vi "VI_X.vi"() -> ()   [LabVIEW 2015]
uses:
  <vilib>/vision/Vision Builder AI/API.llb/IVB Interface - VBAI Version.ctl
panel:
  out "COMMENTS":string
  in  "TOTAL NUMBER OF BRANCHS":i16=16
  out "INSPECTED IMAGE":T1(plugin-control)
  out "STATE TEST":bool
  out "INSPECTION NAME":string
  in  "error in 2":errorcluster
  out "error out 2":errorcluster
  out "INSPECTION PATH":path
  in  "ACTION":T2(ring)
  out "SESSION NAME":string
  in  "Number of Branch X":i16 caption="NUMBER OF BRANCH X" min=0
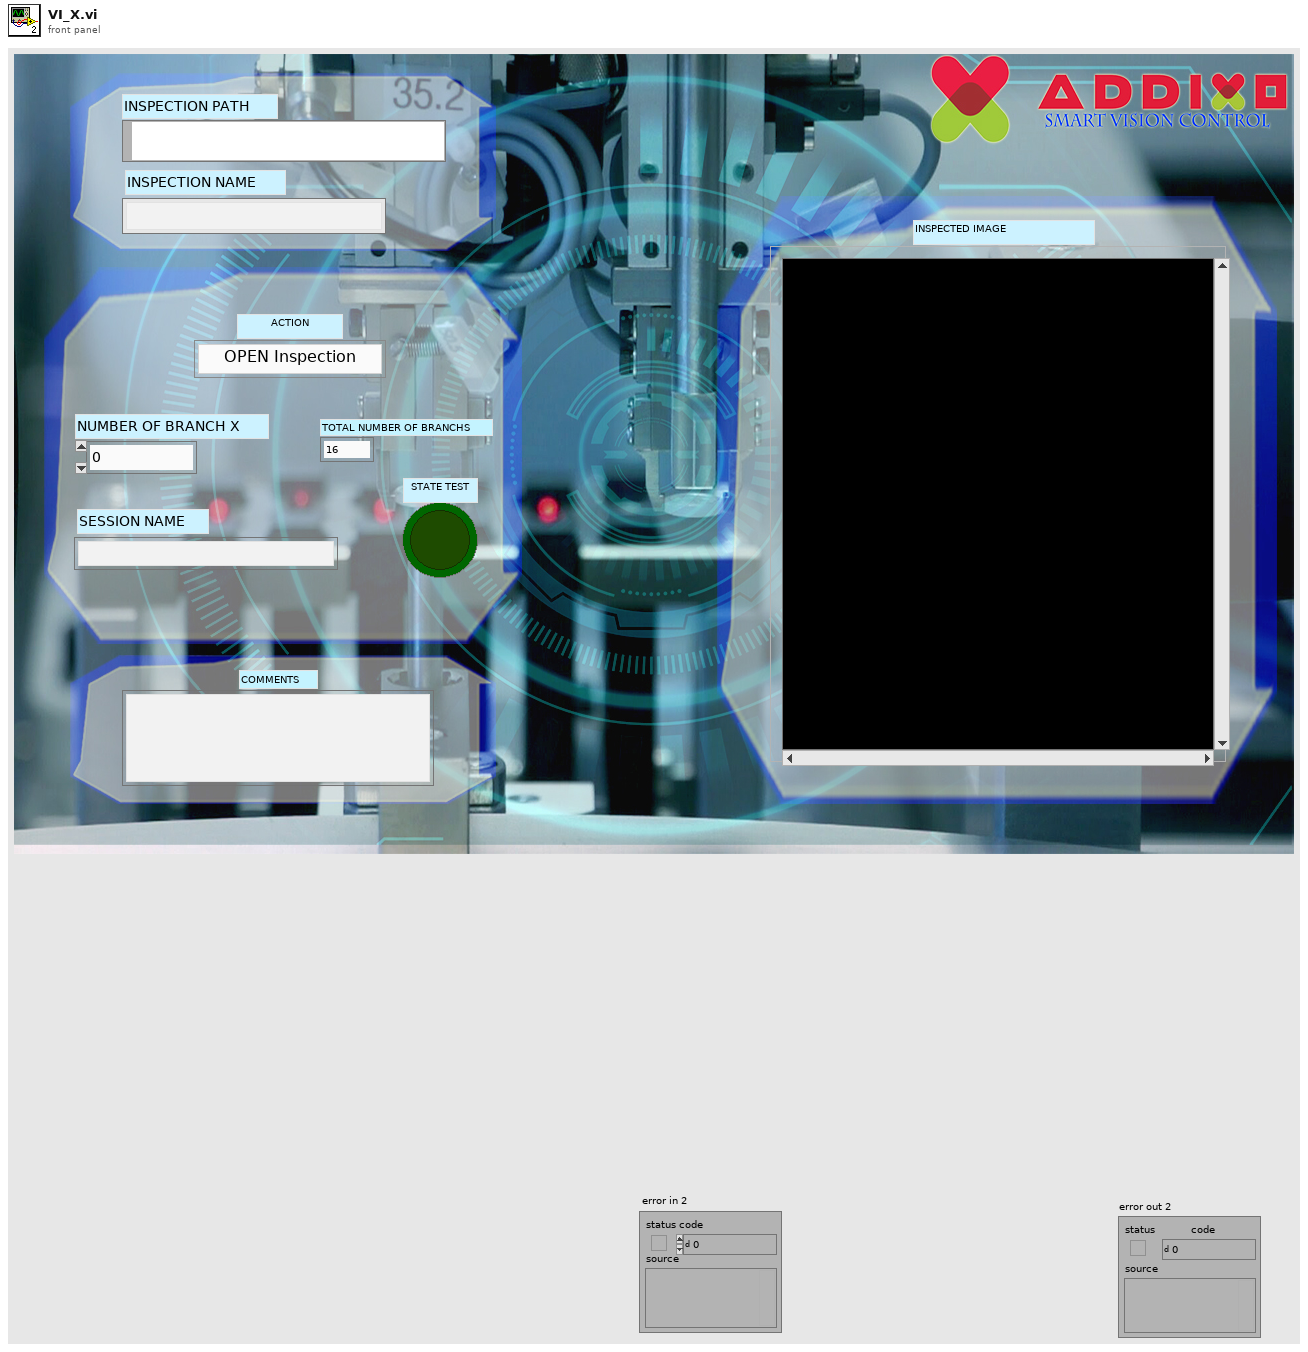
[diagram p1: front panel]
types:
  T1 = typedef "IMAQ Image.ctl" = refnum<image>
  T2 = enum16{"OPEN Inspection", "START Inspection", "Inspect", "CLOSE Inspection"}
  T3 = cluster{"PASS/FAIL Flag":bool, "Numeric Measurement":dbl, "String Measurement":string, "Report Text":string}
  T4 = typedef "IVB Interface - VBAI Version.ctl" = u16
  T5 = typedef "VBAIInterface.ctl" = refnum<k21>
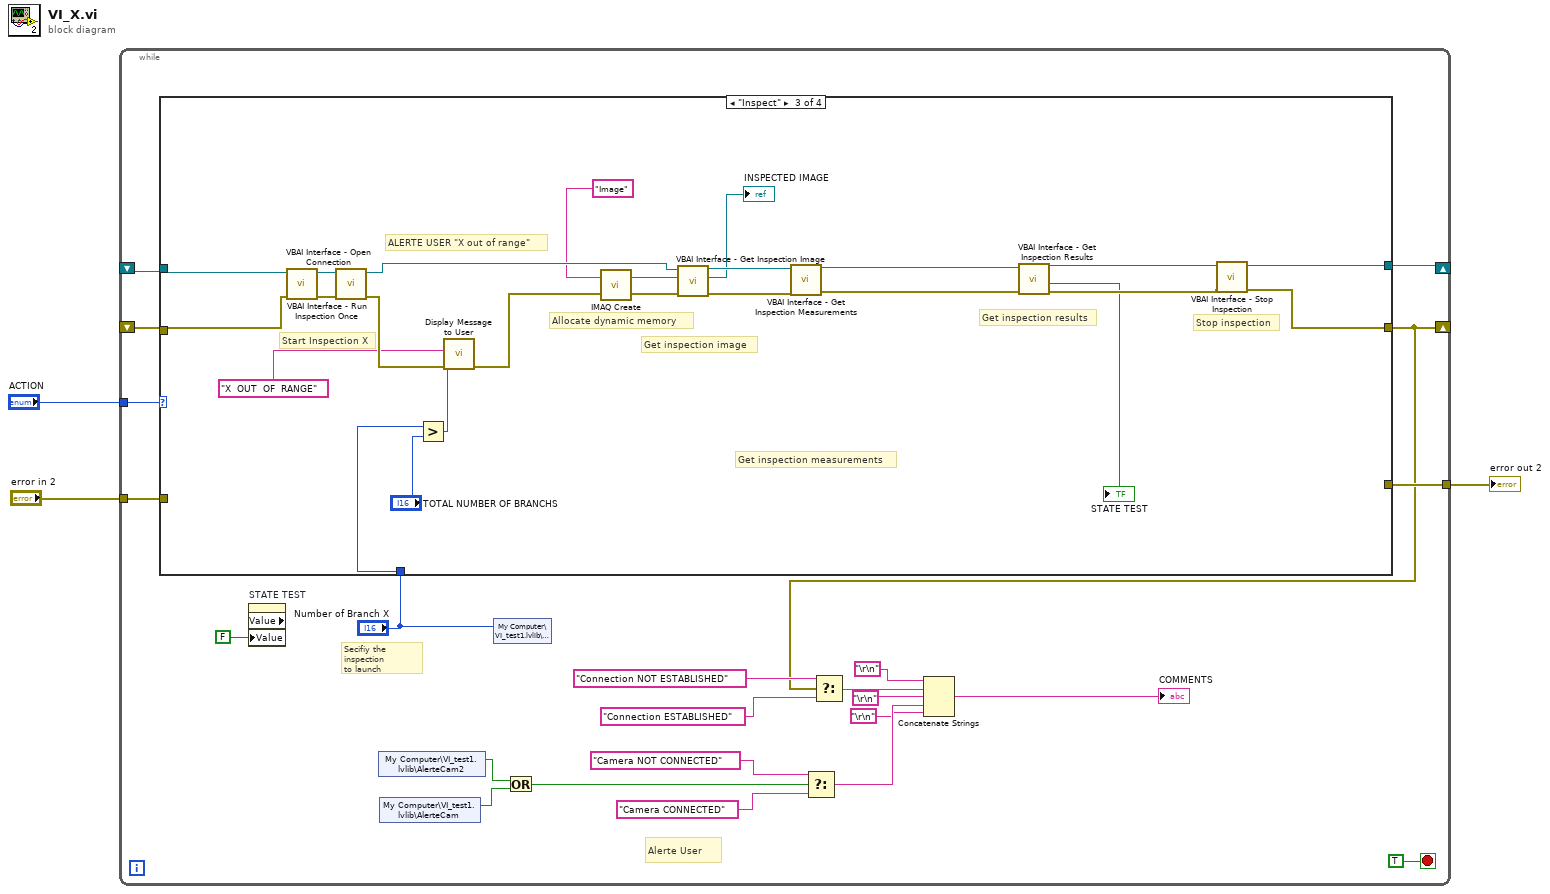
[diagram p0: block diagram]
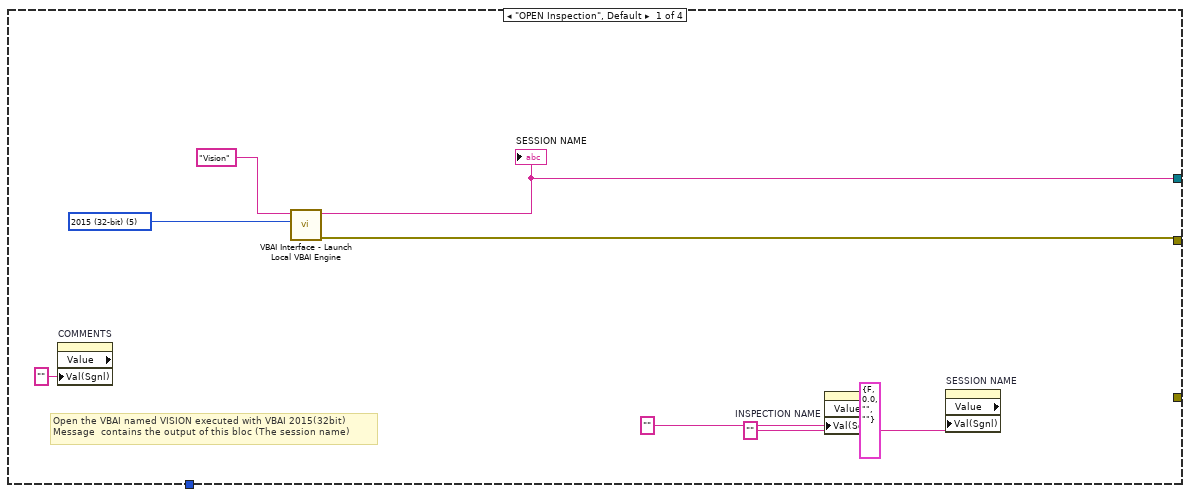
[diagram p2: hidden frame]
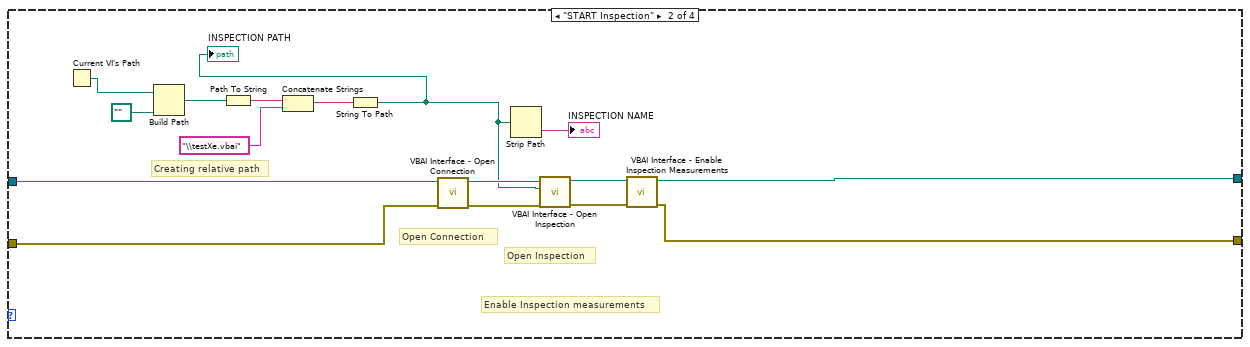
[diagram p3: hidden frame]
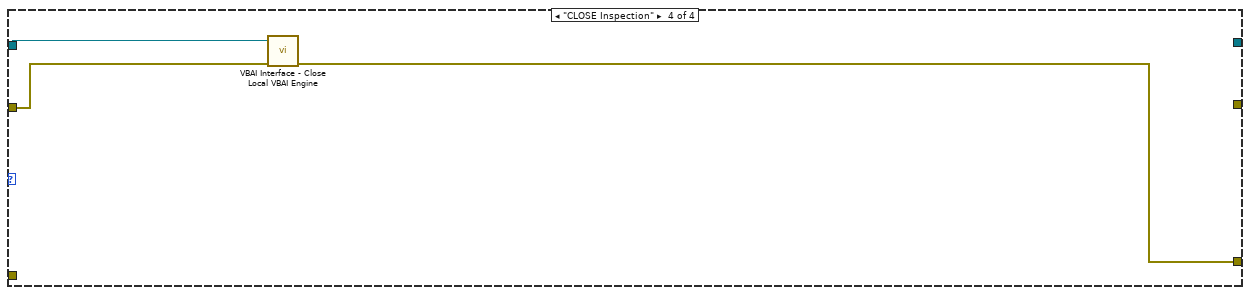
[diagram p4: hidden frame]
diagram:
  n1 = while {
    tunnel: "ACTION" -> [w26]
    shift-right: [w25] -> _
    shift-left: _ -> [w24]
    tunnel: [w23] -> w2
    shift-right: [w9] -> _
    shift-left: _ -> [w22]
    tunnel: "error in 2" -> [w21]
    stop <- TRUE stop-if-true
    # "Alerte User"
    # "Secifiy the inspection \nto launch"
    n2 = case shown="\"Inspect\"" w26 {
      tunnel: [w31 w42 w66 _] -> w25
      tunnel: w24 -> [_ w49 w63 w76]
      tunnel: [_ _ _ w75] -> w23
      tunnel: [w28 w41 w60 _] -> w9
      tunnel: w22 -> [_ w46 w62 w74]
      tunnel: w21 -> [_ _ _ _]
      tunnel: "Number of Branch X" -> [_ _ w52 _]
      frame "OPEN Inspection", Default {
        (unwired) T3 {"PASS/FAIL Flag"=FALSE, "Numeric Measurement"=0.0, "String Measurement"="", "Report Text"=""} ("Value (Signaling)")
        w33 = T4 5 items=["2010 (32-bit)"=0, "2011 (32-bit)"=1, "2012 (32-bit)"=2, "2013 (32-bit)"=3, "2014 (32-bit)"=4, "2014 (64-bit)"=1004, "2015 (32-bit)"=5, "2015 (64-bit)"=1005] ("Engine Version")
        # "Open the VBAI named VISION executed with VBAI 2015(32bit)\nMessage  contains the output of this bloc (The session name)"
        n3 = property on="COMMENTS" class="Str" props=["Value", "Val(Sgnl)"]("Val(Sgnl)"="" ("Value (Signaling)")) -> ()  [unwired: 2 in, 3 out]
        n4 = call <vilib>:"VBAI Interface - Launch Local VBAI Engine.vi"("Engine Version"=w33, "Local VBAI Engine Name"="Vision") -> ("error out"=w28:errorcluster, "Session Name Out"=w31:string)  [unwired: 8 in]
        "SESSION NAME" <- w31
        n5 = property on="INSPECTION NAME" class="Str" props=["Value", "Val(Sgnl)"]("Val(Sgnl)"="" ("Value (Signaling)")) -> ()  [unwired: 2 in, 3 out]
        n6 = property on="SESSION NAME" class="Str" props=["Value", "Val(Sgnl)"]("Val(Sgnl)"="" ("Value (Signaling)")) -> ()  [unwired: 2 in, 3 out]
      }
      frame "START Inspection" {
        # "Creating relative path"
        # "Enable Inspection measurements"
        # "Open Inspection"
        # "Open Connection"
        n7 = Current VI's Path() -> (path=w39:path)
        n8 = Build Path(base path=w39, name or relative path=path "..") -> (appended path=w38:path)
        n9 = Path To String(path=w38) -> (string=w37:string)
        n10 = Concatenate Strings(w37, "\\testXe.vbai" ("string")) -> (w35:string)
        n11 = String To Path(string=w35) -> (path=w34:path)
        "INSPECTION PATH" <- w34
        n12 = call <vilib>:"VBAI Interface - Open Connection.vi"("error in"=w46, "Session In"=w49) -> ("error out"=w48:errorcluster, "Session Out"=w47:T5)  [unwired: 8 in]
        n13 = Strip Path(path=w34) -> (name=→"INSPECTION NAME":string)  [unwired: 1 out]
        n14 = call <vilib>:"VBAI Interface - Open Inspection.vi"("error in"=w48, "Path"=w34, "Session In"=w47) -> ("error out"=w43:errorcluster, "Session Out"=w44:T5)  [unwired: 7 in]
        n15 = call <vilib>:"VBAI Interface - Enable Inspection Measurements.vi"("error in"=w43, "Session In"=w44) -> ("error out"=w41:errorcluster, "Session Out"=w42:T5)  [unwired: 8 in]
      }
      frame "Inspect" {
        # "ALERTE USER \"X out of range\""
        # "Stop inspection"
        # "Get inspection results"
        # "Get inspection measurements"
        # "Get inspection image"
        # "Allocate dynamic memory"
        # "Start Inspection X"
        n16 = call <vilib>:"VBAI Interface - Open Connection.vi"("error in"=w62, "Session In"=w63) -> ("error out"=w64:errorcluster, "Session Out"=w65:T5)  [unwired: 8 in]
        n17 = call <vilib>:"VBAI Interface - Run Inspection Once.vi"("error in"=w64, "Session In"=w65) -> ("error out"=w55:errorcluster, "Session Out"=w73:T5)  [unwired: 8 in]
        n18 = Greater?(x=w52, y="TOTAL NUMBER OF BRANCHS") -> (0:w51:bool)
        n19 = call "Display Message to User"("error in (no error)"=w55, "Enable"=w51, "Message"="X  OUT  OF  RANGE") -> ("error out"=w54:errorcluster)  [unwired: 7 in, 1 out]
        n20 = call "IMAQ Create"("Image Name"="Image", "error in (no error)"=w54) -> ("New Image"=w61:T1, "error out"=w68:errorcluster)  [unwired: 3 in]
        n21 = call <vilib>:"VBAI Interface - Get Inspection Image.vi"("error in"=w68, "Image Dest"=w61, "Session In"=w73) -> ("error out"=w72:errorcluster, "Image Dst Out"=→"INSPECTED IMAGE":T1, "Session Out"=w71:T5)  [unwired: 5 in, 1 out]
        n22 = call <vilib>:"VBAI Interface - Get Inspection Measurements.vi"("error in"=w72, "Session In"=w71) -> ("error out"=w69:errorcluster, "Session Out"=w70:T5)  [unwired: 4 in, 4 out]
        n23 = call <vilib>:"VBAI Interface - Get Inspection Results.vi"("error in"=w69, "Session In"=w70) -> ("error out"=w58:errorcluster, "Inspection Status"=→"STATE TEST":bool, "Session Out"=w59:T5)  [unwired: 3 in, 4 out]
        n24 = call <vilib>:"VBAI Interface - Stop Inspection.vi"("error in"=w58, "Session In"=w59) -> ("error out"=w60:errorcluster, "Session Out"=w66:T5)  [unwired: 8 in]
      }
      frame "CLOSE Inspection" {
        n25 = call <vilib>:"VBAI Interface - Close Local VBAI Engine.vi"("error in"=w74, "Session Name In"=w76) -> ("error out"=w75:errorcluster)  [unwired: 9 in]
      }
    }
    n26 = property on="STATE TEST" class="Bool (strict)" props=["Value", "Value"]("Value"=FALSE ("Value (Signaling)")) -> ()  [unwired: 2 in, 3 out]
    n27 = shared-variable "My Computer\\VI_test1.lvlib\\AlerteCam2"() -> (w7:bool)  [unwired: 1 in, 1 out]
    n28 = shared-variable "My Computer\\VI_test1.lvlib\\AlerteCam"() -> (w6:bool)  [unwired: 1 in, 1 out]
    n29 = shared-variable "My Computer\\VI_test1.lvlib\\Xe"("Number of Branch X") -> ()  [unwired: 1 in, 1 out]
    n30 = Or(x=w7, y=w6) -> (x .or. y?=w5:bool)
    n31 = Select(t="Camera NOT CONNECTED" ("Message"), s=w5, f="Camera CONNECTED" ("Message")) -> (s? t:f=w12:string)
    n32 = Select(t="Connection NOT ESTABLISHED" ("Message"), s=w9, f="Connection ESTABLISHED" ("Message")) -> (s? t:f=w14:string)
    n33 = Concatenate Strings("\r\n", w14, "\r\n", w12, "\r\n") -> (→"COMMENTS":string)
  }
  "error out 2" <- w2
